vi "Get Section.vi"(8 "error in":errorcluster, 11 "Object Entry in":refnum<class "Section.lvclass">) -> (0 "error out":errorcluster, 2 "Section":string, 3 "Object Entry out":refnum<class "Section.lvclass">)   [LabVIEW 2024, in "EDS.lvlib" / "Section.lvclass"]
uses:
  Section.lvclass
  Section.lvclass/Section.ctl
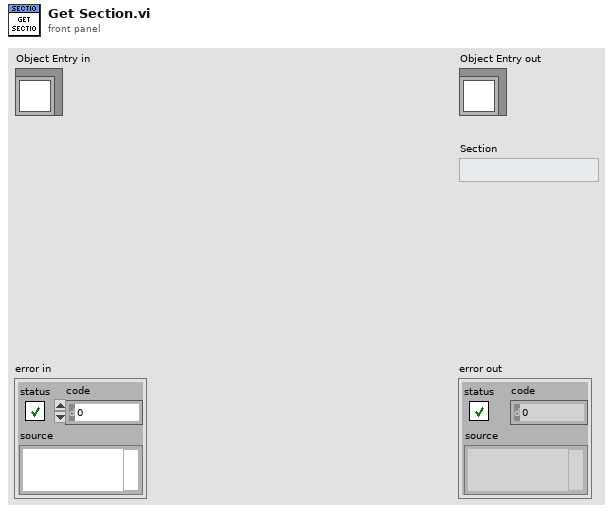
[diagram p1: front panel]
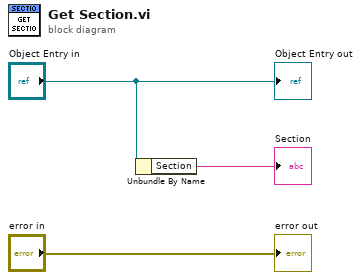
[diagram p0: block diagram]
diagram:
  n1 = Unbundle By Name("Object Entry in") -> ("Section"=→"Section":string)
  "error out" <- "error in"
  "Object Entry out" <- "Object Entry in"
